vi "Temp.vi"() -> ()   [LabVIEW 2018]
panel:
  in  "Boolean 10":bool
  in  "Boolean 9":bool
  in  "Boolean 8":bool
  in  "Boolean 7":bool
  in  "Boolean 6":bool
  in  "Boolean 5":bool
  in  "Table Control 2":string[][](table)
  in  "Table Control":string[][](table)
  in  "Boolean 4":bool
  in  "Boolean 3":bool
  in  "Boolean 2":bool
  in  "Boolean":bool
  # "BMS Monitor"
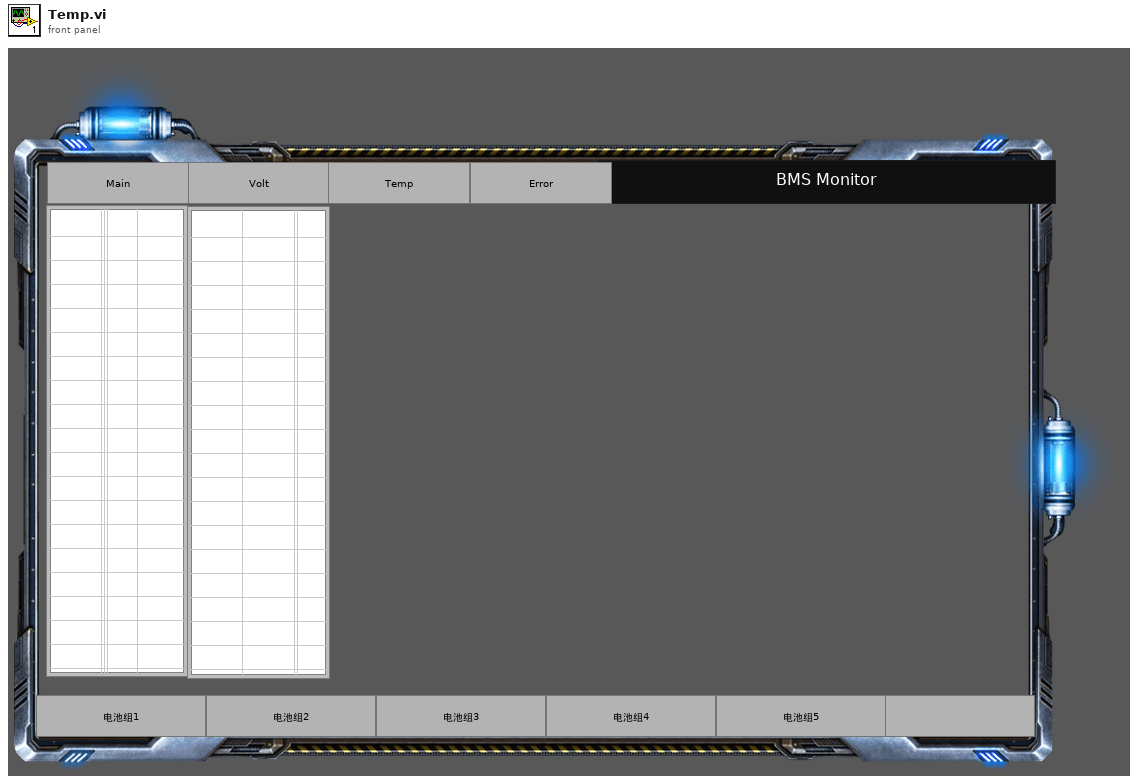
[diagram p1: front panel]
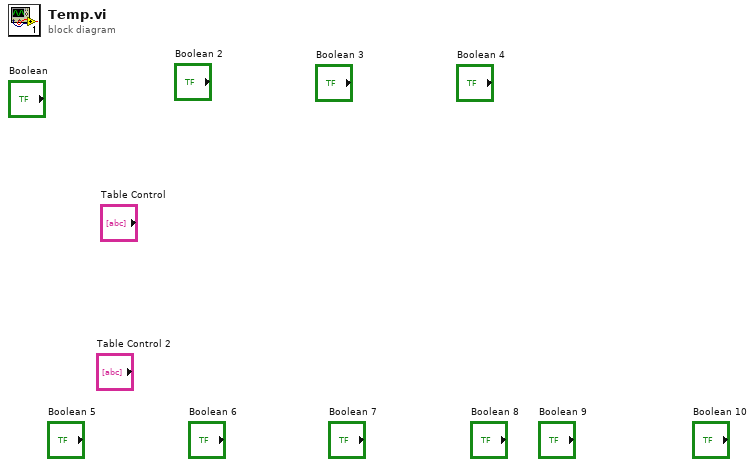
[diagram p0: block diagram]
diagram:
